vi "SRV_Parse Response (QR Code).vi"(0 "data":string, 11 "error in (no error)":errorcluster) -> (8 "QR Code":string, 15 "error out":errorcluster)   [LabVIEW 2014]
doc: "Parses a QR Code packet.\n\nIf, and only if, a valid QR tag is seen and decoded, the BFin will send a \"##g:7\" packet. (those will be the first 5 bytes of the payload). After those bytes, there will be a space, a single quote, then the value decoded from the QR tag, and then another single quote. For example, if the QR tag had the data \"Tim Jump Rocks!\" encoded in it, you'd get this packet:\n##g:7 'Tim Jump Rocks!'\n\n\nAuthor: Mike Schultz\nmschultz11711@gmail.com"
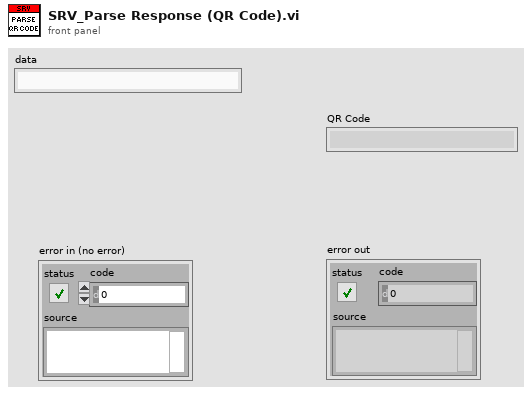
[diagram p1: front panel]
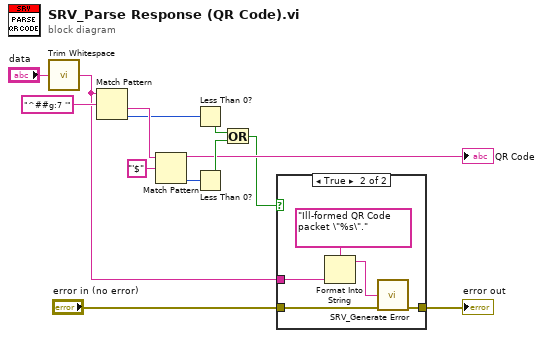
[diagram p0: block diagram]
diagram:
  n1 = call <vilib>:"Trim Whitespace.vi"("string"="data") -> ("trimmed string"=w1:string)  [unwired: 1 in]
  n2 = Match Pattern(string=w1, regular expression="^##g:7 '") -> (after substring=w12:string, offset past match=w10:i32)  [unwired: 1 in, 2 out]
  n3 = Match Pattern(string=w12, regular expression="'$") -> (before substring=→"QR Code":string, offset past match=w9:i32)  [unwired: 1 in, 2 out]
  n4 = Less Than 0?(x=w10) -> (x < 0?=w8:bool)
  n5 = Less Than 0?(x=w9) -> (x < 0?=w7:bool)
  n6 = Or(x=w8, y=w7) -> (x .or. y?=w5:bool)
  n7 = case shown="True" w5 {
    tunnel: "error in (no error)" -> [w14 w17]
    tunnel: [w14 w16] -> w3
    tunnel: w1 -> [_ w15]
    frame False {
    }
    frame True {
      n8 = Format Into String(format string="Ill-formed QR Code packet \"%s\".", w15) -> (resulting string=w18:string)  [unwired: 2 in, 1 out]
      n9 = call "SRV_Generate Error.vi"("Message"=w18, "error in (no error)"=w17) -> ("error out"=w16:errorcluster)  [unwired: 13 in]
    }
  }
  "error out" <- w3
